vi "coord calculate.vi"(9 "theta":dbl format="%#_13g", 10 "coord in":cdb format="%#_13g", 11 "pieceOfWorld in":T1[][](array[typedef])) -> (1 "length":dbl, 2 "coord out":cdb)   [LabVIEW 2015, in "PolyVIEW.lvclass"]
uses:
  PolyVIEW.lvclass
  actors/world/typedefs/worldCell_cluster.ctl
  actors/world/typedefs/markValue_cluster.ctl
  actors/world/typedefs/markValue.ctl
  actors/world/typedefs/markVolume.ctl
  actors/world/typedefs/amountOfFood.ctl
  actors/world/typedefs/anthillType_enum.ctl
  classes/altitudes/altitudes_layer.lvclass
  actors/world/world.lvlib
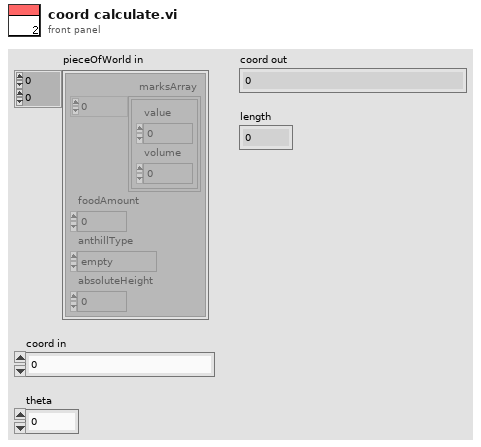
[diagram p1: front panel]
types:
  T1 = typedef "world.lvlib/worldCell_cluster.ctl" = cluster{"marksArray":T2[], "foodAmount":T5, "anthillType":T6, "absoluteHeight":u8}
  T2 = typedef "world.lvlib/markValue_cluster.ctl" = cluster{"value":T3, "volume":T4}
  T3 = typedef "world.lvlib/markValue.ctl" = u8
  T4 = typedef "world.lvlib/markVolume.ctl" = u16
  T5 = typedef "world.lvlib/amountOfFood.ctl" = i32
  T6 = typedef "world.lvlib/anthillType_enum.ctl" = enum16{"empty", "own", "rival"}
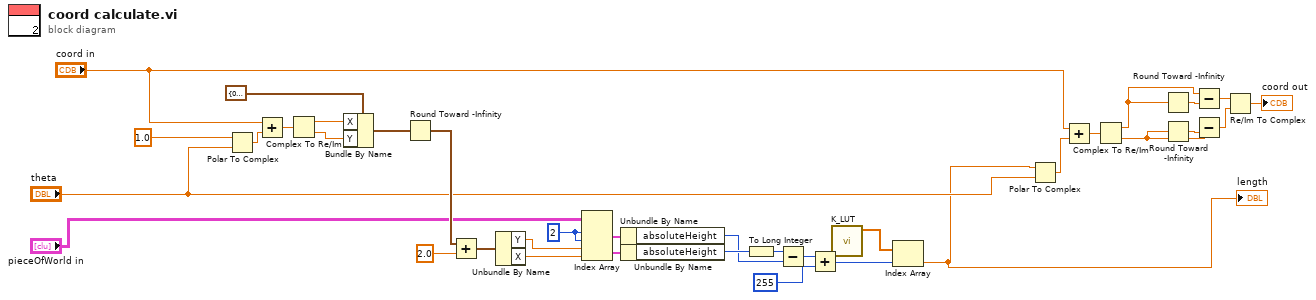
[diagram p0: block diagram]
diagram:
  w14 = 2 ("index (row)")
  n1 = Polar To Complex(1:"theta", 2:1.0 ("r")) -> (0:w7:cdb)
  n2 = Add(x="coord in", y=w7) -> (x+y=w4:cdb)
  n3 = Complex To Re/Im(x + iy=w4) -> (x=w5:dbl, y=w6:dbl)
  n4 = Bundle By Name(cluster=cluster{"X":dbl, "Y":dbl} {"X"=0.0, "Y"=0.0} ("pointIn"), "X"=w5, "Y"=w6) -> (w12:cluster{"X":dbl, "Y":dbl})
  n5 = Round Toward -Infinity(1:w12) -> (0:w15:cluster{"X":dbl, "Y":dbl})
  n6 = Add(x=w15, y=2.0) -> (x+y=w17:cluster{"X":dbl, "Y":dbl})
  n7 = Unbundle By Name(w17) -> ("Y"=w13:dbl, "X"=w18:dbl)
  n8 = Index Array(array="pieceOfWorld in", index (row) #1=w14, index (col) #1=w14, index (row) #2=w13, index (col) #2=w18) -> (element #1=w19:T1, element #2=w20:T1)
  n9 = Unbundle By Name(w19) -> ("absoluteHeight"=w26:u8)
  n10 = Unbundle By Name(w20) -> ("absoluteHeight"=w27:u8)
  n11 = To Long Integer(number=w27) -> (32bit integer=w21:i32)
  n12 = Subtract(x=w21, y=w26) -> (x-y=w22:i32)
  n13 = Add(x=w22, y=255) -> (x+y=w25:i32)
  n14 = call "K_LUT.vi"() -> ("K-LUT"=w24:dbl[])  [unwired: 11 in]
  n15 = Index Array(array=w24, index=w25) -> (element=w2:dbl)
  "length" <- w2
  n16 = Polar To Complex(1:"theta", 2:w2) -> (0:w8:cdb)
  n17 = Add(x="coord in", y=w8) -> (x+y=w34:cdb)
  n18 = Complex To Re/Im(x + iy=w34) -> (x=w28:dbl, y=w31:dbl)
  n19 = Round Toward -Infinity(1:w28) -> (0:w29:dbl)
  n20 = Round Toward -Infinity(1:w31) -> (0:w30:dbl)
  n21 = Subtract(x=w28, y=w29) -> (x-y=w32:dbl)
  n22 = Subtract(x=w31, y=w30) -> (x-y=w33:dbl)
  n23 = Re/Im To Complex(1:w33, 2:w32) -> (0:→"coord out":cdb)
